vi "Filter Event Data.vi"(8 "error in (no error)":errorcluster, 10 "EventFilter Reference":T1, 11 "ControlDragOverMsg In":refnum<class "ControlDragOverMsg.lvclass">) -> (0 "error out":errorcluster, 2 "Discard?":bool, 3 "ControlDragOverMsg Out":refnum<class "ControlDragOverMsg.lvclass">)   [LabVIEW 2017, in "ActorEvents.lvlib" / "ControlDragOverMsg.lvclass"]
uses:
  ControlDragOverMsg.lvclass
  IEventFilter/EventFilter Reference.ctl
  IEventFilter/IEventFilter.lvclass
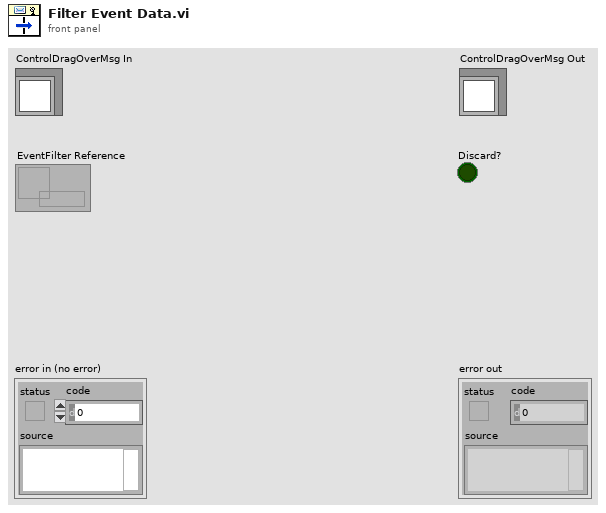
[diagram p1: front panel]
types:
  T1 = typedef "ActorEvents.lvlib/IEventFilter.lvclass/EventFilter Reference.ctl" = refnum<data-value>
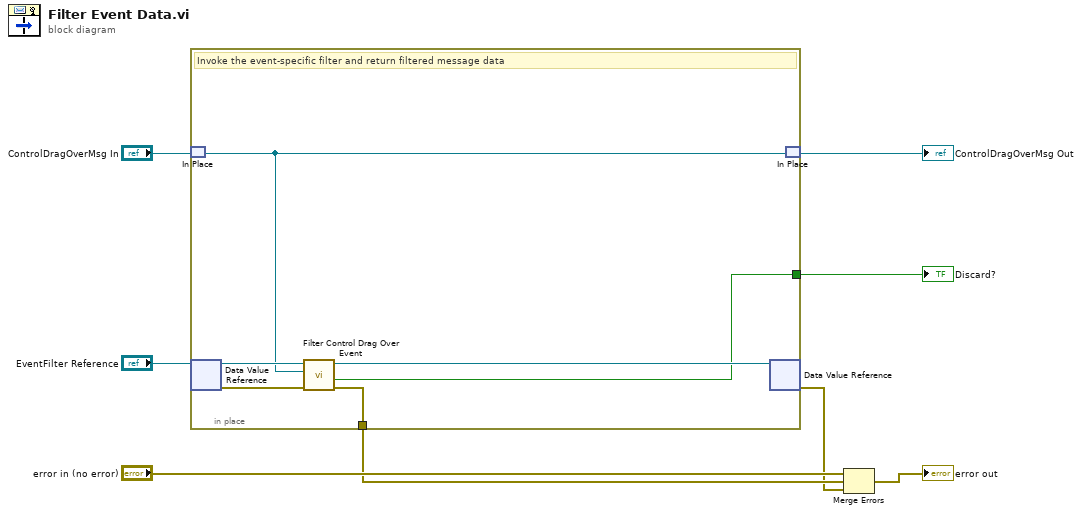
[diagram p0: block diagram]
diagram:
  n1 = in-place {
    in-place-border: [w10] -> w5
    in-place-border: [w11] -> w3
    # "Invoke the event-specific filter and return filtered message data"
    n2 = in-place-match #1("ControlDragOverMsg In") -> (w9:refnum<class "ControlDragOverMsg.lvclass">)
    n3 = in-place-dvr #2("EventFilter Reference") -> (w14:refnum<class "IEventFilter.lvclass">, w12:errorcluster)
    n4 = call-dynamic "Filter Control Drag Over Event.vi"("error in (no error)"=w12, "ControlDragOverMsg"=w9, "IEventFilter in"=w14) -> ("error out"=w10:errorcluster, "Discard?"=w11:bool, "IEventFilter out"=w13:refnum<class "IEventFilter.lvclass">)  [unwired: 6 in]
    n5 = in-place-dvr #2(w13) -> (w4:errorcluster)  [unwired: 1 out]
    n6 = in-place-match #1(w9) -> (→"ControlDragOverMsg Out":refnum<class "ControlDragOverMsg.lvclass">)
  }
  "Discard?" <- w3
  n7 = Merge Errors("error in (no error)", w5, w4) -> (→"error out":errorcluster)
